vi "Check Last Publish.vi"(8 "error in (no error)":errorcluster, 11 "Log Manager Module in":refnum<class "Log Manager Module.lvclass">) -> (0 "error out":errorcluster, 3 "Log Manager Module out":refnum<class "Log Manager Module.lvclass">)   [LabVIEW 2023, in "VolatusData.lvlib" / "Log Manager Module.lvclass"]
uses:
  Log Manager Module.lvclass
  Log Manager Module.lvclass/Log Manager Module.ctl
  Volatus/Module/Module.lvclass
  C:/dev/volatus/mts-volatus-super/libs/lv-volatus/Volatus/Module/Module.lvclass
  C:/dev/volatus/mts-volatus-super/libs/lv-volatus/VolatusData/Log Manager Module/Log Manager Module.lvclass
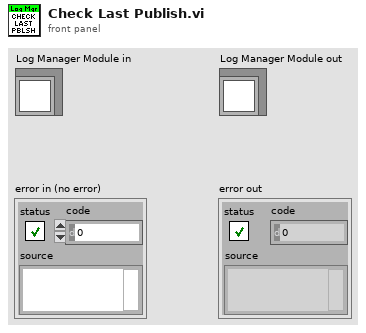
[diagram p1: front panel]
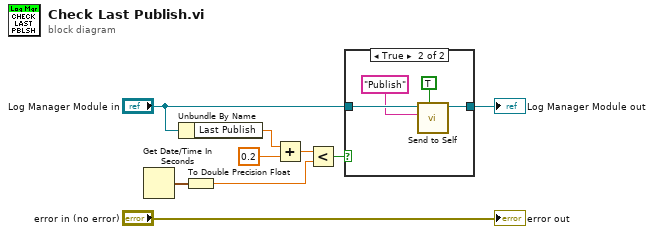
[diagram p0: block diagram]
diagram:
  n1 = Get Date/Time In Seconds() -> (seconds since 1Jan1904=w8:timestamp)
  n2 = Unbundle By Name("Log Manager Module in") -> ("Last Publish"=w7:dbl)
  n3 = To Double Precision Float(number=w8) -> (double precision float=w4:dbl)
  n4 = Add(x=w7, y=0.2) -> (x+y=w5:dbl)
  n5 = Less?(x=w5, y=w4) -> (x < y?=w3:bool)
  n6 = case shown="True" w3 {
    tunnel: "Log Manager Module in" -> [w10 w14]
    tunnel: [w10 w11] -> w1
    frame False {
    }
    frame True {
      n7 = call "Send to Self.vi"("High Priority (F)"=TRUE, "Message ID"="Publish", "Module in"=w14) -> ("Module out"=w11:refnum<class "Log Manager Module.lvclass">)  [unwired: 7 in, 1 out]
    }
  }
  "Log Manager Module out" <- w1
  "error out" <- "error in (no error)"
